vi "Read Expression.vi"(8 "error in (no error)":errorcluster, 11 "muExpr in":refnum<class "muExpr.lvclass">) -> (0 "error out":errorcluster, 2 "Expression":string, 3 "muExpr out":refnum<class "muExpr.lvclass">)   [LabVIEW 2015, in "muParser.lvlib" / "muExpr.lvclass"]
uses:
  muExpr.lvclass
  muExpr.lvclass/muExpr.ctl
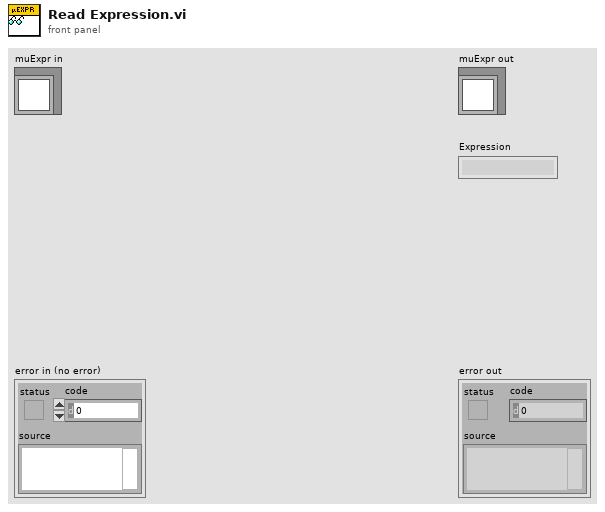
[diagram p1: front panel]
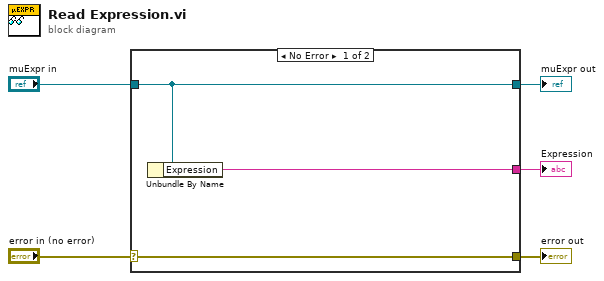
[diagram p0: block diagram]
diagram:
  n1 = case shown="No Error" "error in (no error)" {
    selector: "error in (no error)" -> [w8 w9]
    tunnel: [w8 w9] -> w4
    tunnel: [w7 w10] -> w2
    tunnel: "muExpr in" -> [w7 w10]
    tunnel: [w6 _] -> w1
    frame No Error {
      n2 = Unbundle By Name(w7) -> ("Expression"=w6:string)
    }
    frame Error {
    }
  }
  "error out" <- w4
  "muExpr out" <- w2
  "Expression" <- w1
